vi "SaveFcRecordToFile.vi"(8 "error in (no error)":errorcluster caption="Fehler (Eingang, kein Fehler)", 10 "FC-Data":string[][](array[string])) -> (0 "error out":errorcluster caption="Fehler (Ausgang)")   [LabVIEW 2017]
uses:
  <vilib>/Utility/file.llb/Write To Spreadsheet File (string).vi
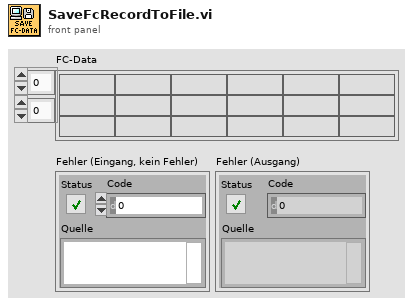
[diagram p1: front panel]
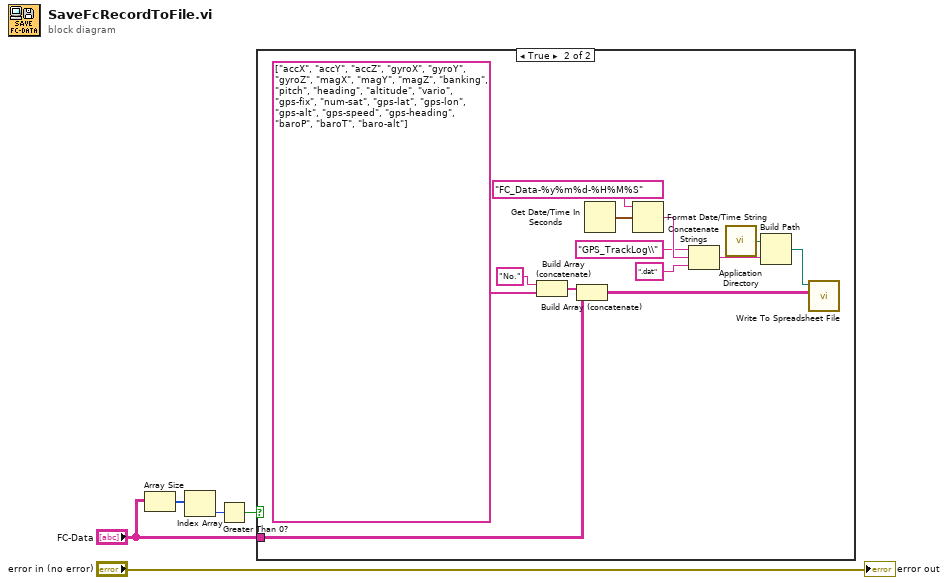
[diagram p0: block diagram]
diagram:
  n1 = Array Size(array="FC-Data") -> (size(s)=w3:i32[])
  n2 = Index Array(array=w3) -> (element=w2:i32)  [unwired: 1 in]
  n3 = Greater Than 0?(x=w2) -> (x > 0?=w1:bool)
  n4 = case shown="True" w1 {
    tunnel: "FC-Data" -> [_ w15]
    frame False {
    }
    frame True {
      n5 = Build Array (concatenate)("No.", string[] ["accX", "accY", "accZ", "gyroX", "gyroY", "gyroZ", "magX", "magY", "magZ", "banking", "pitch", "heading", "altitude", "vario", "gps-fix", "num-sat", "gps-lat", "gps-lon", "gps-alt", "gps-speed", "gps-heading", "baroP", "baroT", "baro-alt"]) -> (w16:string[])
      n6 = Build Array (concatenate)(w16, w15) -> (w11:string[][])
      n7 = Get Date/Time In Seconds() -> (seconds since 1Jan1904=w9:timestamp)
      n8 = Format Date/Time String(time format string (%c)="FC_Data-%y%m%d-%H%M%S" ("Zeitformatierungs-String (%c)"), seconds (now)=w9) -> (date/time string=w7:string)  [unwired: 1 in]
      n9 = Concatenate Strings("GPS_TrackLog\\" ("String"), w7, ".dat" ("String")) -> (w12:string)
      n10 = call <vilib>:"Application Directory.vi"() -> ("Application Directory"=w14:path)
      n11 = Build Path(base path=w14, name or relative path=w12) -> (appended path=w10:path)
      n12 = call-poly <vilib>:"Write To Spreadsheet File.vi"("2D data"=w11, "file path (dialog if empty)"=w10) -> ()  [unwired: 6 in, 1 out]
    }
  }
  "error out" <- "error in (no error)"
